vi "isChannelInScript.vi"(8 "error in (no error)":errorcluster, 10 "channelName":string, 11 "ScriptEventList in":refnum<class "ScriptEventList.lvclass">) -> (0 "error out":errorcluster, 2 "found Channel":bool, 3 "ScriptEventList out":refnum<class "ScriptEventList.lvclass">)   [LabVIEW 2011, in "Tools.lvlib" / "Scripting.lvlib" / "ScriptEventList.lvclass"]
uses:
  ScriptEventList.lvclass
  ScriptEventList.lvclass/ScriptEventList.ctl
  ScriptEvent.lvclass
  DatabaseHelpers/Database Objects/Channel/Channel.lvclass
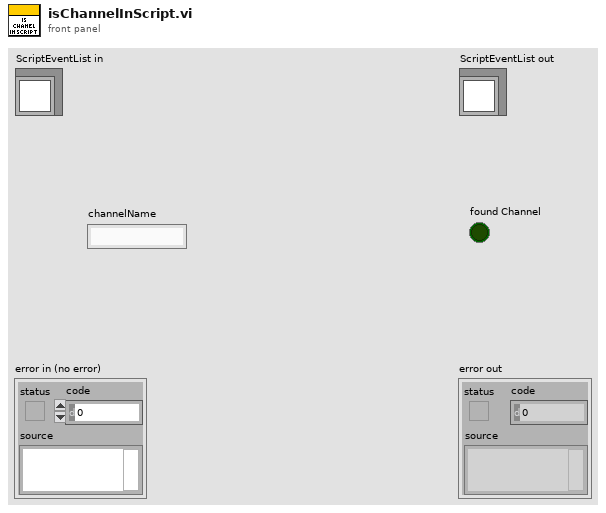
[diagram p1: front panel]
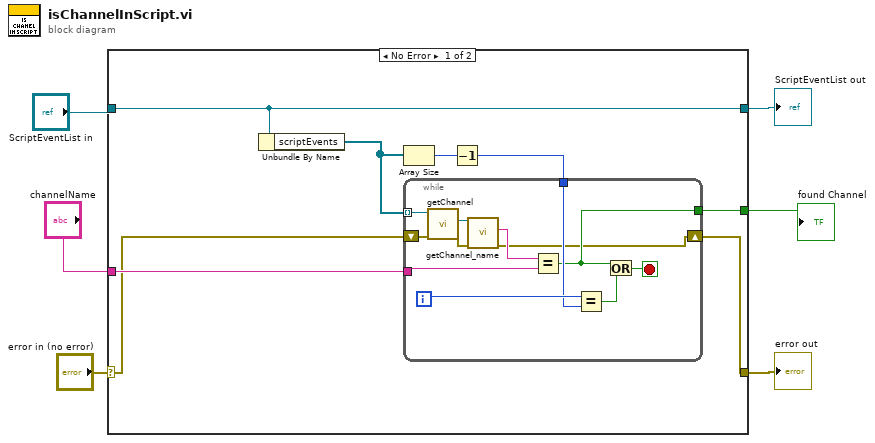
[diagram p0: block diagram]
diagram:
  n1 = case shown="No Error" "error in (no error)" {
    selector: "error in (no error)" -> [w9 w28]
    tunnel: [w8 w28] -> w5
    tunnel: [w14 w27] -> w3
    tunnel: "ScriptEventList in" -> [w14 w27]
    tunnel: "channelName" -> [w13 _]
    tunnel: [w7 _] -> w1
    frame No Error {
      n2 = Unbundle By Name(w14) -> ("scriptEvents"=w12:refnum<class "ScriptEvent.lvclass">[])
      n3 = Array Size(array=w12) -> (size(s)=w11:i32)
      n4 = Decrement(x=w11) -> (x-1=w10:i32)
      n5 = while {
        tunnel: w12 -> [w26] mode=indexing
        tunnel: w13 -> [w22]
        shift-right: [w15] -> w8
        shift-left: w9 -> [w16]
        tunnel: w10 -> [w20]
        tunnel: [w17] -> w7
        i -> [w21]
        stop <- w18 stop-if-true
        n6 = call-dynamic "getChannel.vi"("error in (no error)"=w16, "ScriptEvent.lvclass in"=w26) -> ("error out"=w24:errorcluster, "Channel.lvclass"=w25:refnum<class "Channel.lvclass">)  [unwired: 7 in, 1 out]
        n7 = call "getChannel_name.vi"("error in (no error)"=w24, "Channel.lvclass in"=w25) -> ("error out"=w15:errorcluster, "channel_name"=w23:string)  [unwired: 7 in, 1 out]
        n8 = Equal?(x=w23, y=w22) -> (x = y?=w17:bool)
        n9 = Equal?(x=w21, y=w20) -> (x = y?=w19:bool)
        n10 = Or(x=w17, y=w19) -> (x .or. y?=w18:bool)
      }
    }
    frame Error {
    }
  }
  "error out" <- w5
  "ScriptEventList out" <- w3
  "found Channel" <- w1
